vi "getData.vi"(8 "error in (no error)":errorcluster, 11 "AnalogOutput.lvclass in":refnum<class "AnalogOutput.lvclass">) -> (0 "error out":errorcluster, 2 "Data":dbl[][](array[numeric]), 3 "AnalogOutput.lvclass out":refnum<class "AnalogOutput.lvclass">)   [LabVIEW 2009, in "Hardware.lvlib" / "Channels.lvlib" / "AnalogOutput.lvclass"]
uses:
  AnalogOutput.lvclass
  AnalogOutput.lvclass/AnalogOutput.ctl
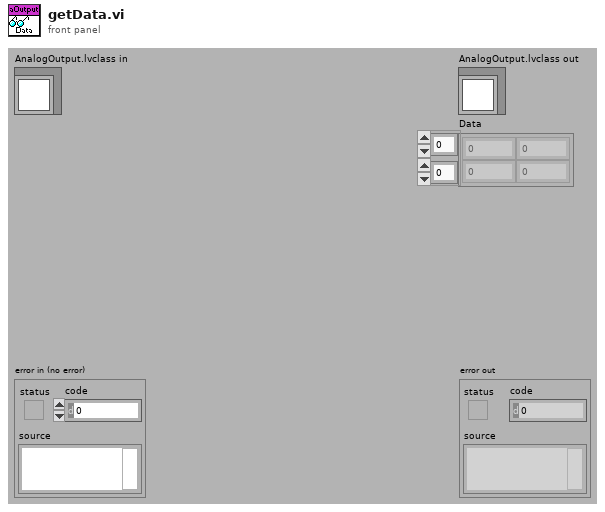
[diagram p1: front panel]
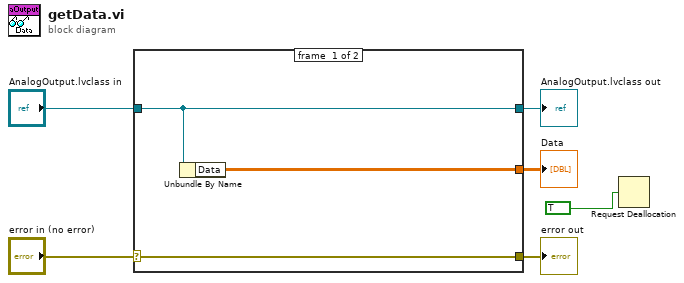
[diagram p0: block diagram]
diagram:
  n1 = case shown="No Error" "error in (no error)" {
    selector: "error in (no error)" -> [w9 w10]
    tunnel: [w9 w10] -> w5
    tunnel: [w8 w11] -> w3
    tunnel: "AnalogOutput.lvclass in" -> [w8 w11]
    tunnel: [w7 _] -> w2
    frame #0 {
      n2 = Unbundle By Name(w8) -> ("Data"=w7:dbl[][])
    }
    frame #1 {
    }
  }
  "error out" <- w5
  "AnalogOutput.lvclass out" <- w3
  "Data" <- w2
  n3 = Request Deallocation(TRUE) -> ()
